vi "Read Message Array.vi"(8 "error in (no error)":errorcluster, 11 "Batch Msg in":refnum<class "Batch Msg.lvclass">) -> (0 "error out":errorcluster, 2 "Message Array":refnum<class "Message.lvclass">[](array[class]), 3 "Batch Msg out":refnum<class "Batch Msg.lvclass">)   [LabVIEW 2020, in "Sequencer.lvlib" / "Batch Msg.lvclass"]
doc: "Read Message Array from the Batch Msg class."
uses:
  Batch Msg.lvclass
  PPL/HDH.Actor Framework.Core.Actor.lvlibp/1abvi3w/vi.lib/ActorFramework/Message/Message.lvclass
  Batch Msg.lvclass/Batch Msg.ctl
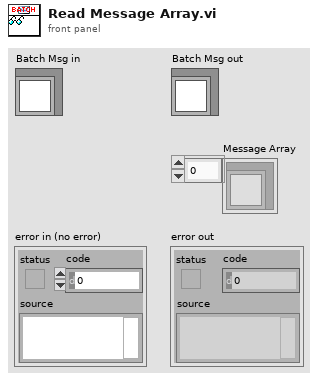
[diagram p1: front panel]
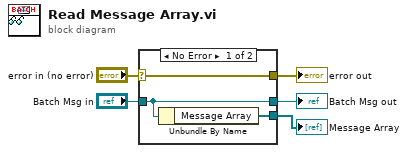
[diagram p0: block diagram]
diagram:
  n1 = case shown="No Error" "error in (no error)" {
    selector: "error in (no error)" -> [w8 w9]
    tunnel: [w8 w9] -> w4
    tunnel: [w7 w10] -> w2
    tunnel: "Batch Msg in" -> [w7 w10]
    tunnel: [w6 _] -> w1
    frame No Error {
      n2 = Unbundle By Name(w7) -> ("Message Array"=w6:refnum<class "Message.lvclass">[])
    }
    frame Error {
    }
  }
  "error out" <- w4
  "Batch Msg out" <- w2
  "Message Array" <- w1
